vi "example_01_table_scrollbars.vi"() -> ()   [LabVIEW 2015, in "lv-pagination.lvlib"]
doc: "This example shows how to use both auto-sizing AND paging with a static data set that can be changed at will."
uses:
  lv-pagination.lvlib
  public/_controls/configuratin_resize.ctl
panel:
  in  "actual_fuzzy":bool
  in  "random":bool
  in  "configuration":T1=enum."all"
  in  "precision":i32=6
  out "configuration []":cluster{"width":u32, "height":u32}[](array[cluster])
  in  "rows":i32=100
  in  "columns":i32=20
  in  "auto_size":bool
  in  "load_column_width":bool
  in  "save_column_width":bool
  in  "sticky_column":i32=-1
  out "data":i32(listbox)=-1
  in  "horizontal":i32(c297)
  in  "vertical":i32(c297)
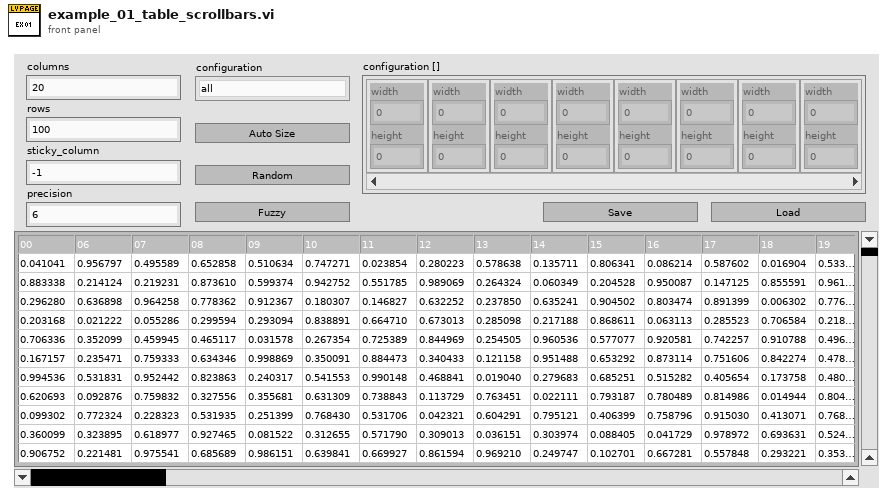
[diagram p1: front panel]
types:
  T1 = typedef "lv-pagination.lvlib/configuratin_resize.ctl" = enum16{"<resize_config>", "header", "contents", "all", "best_fit"}
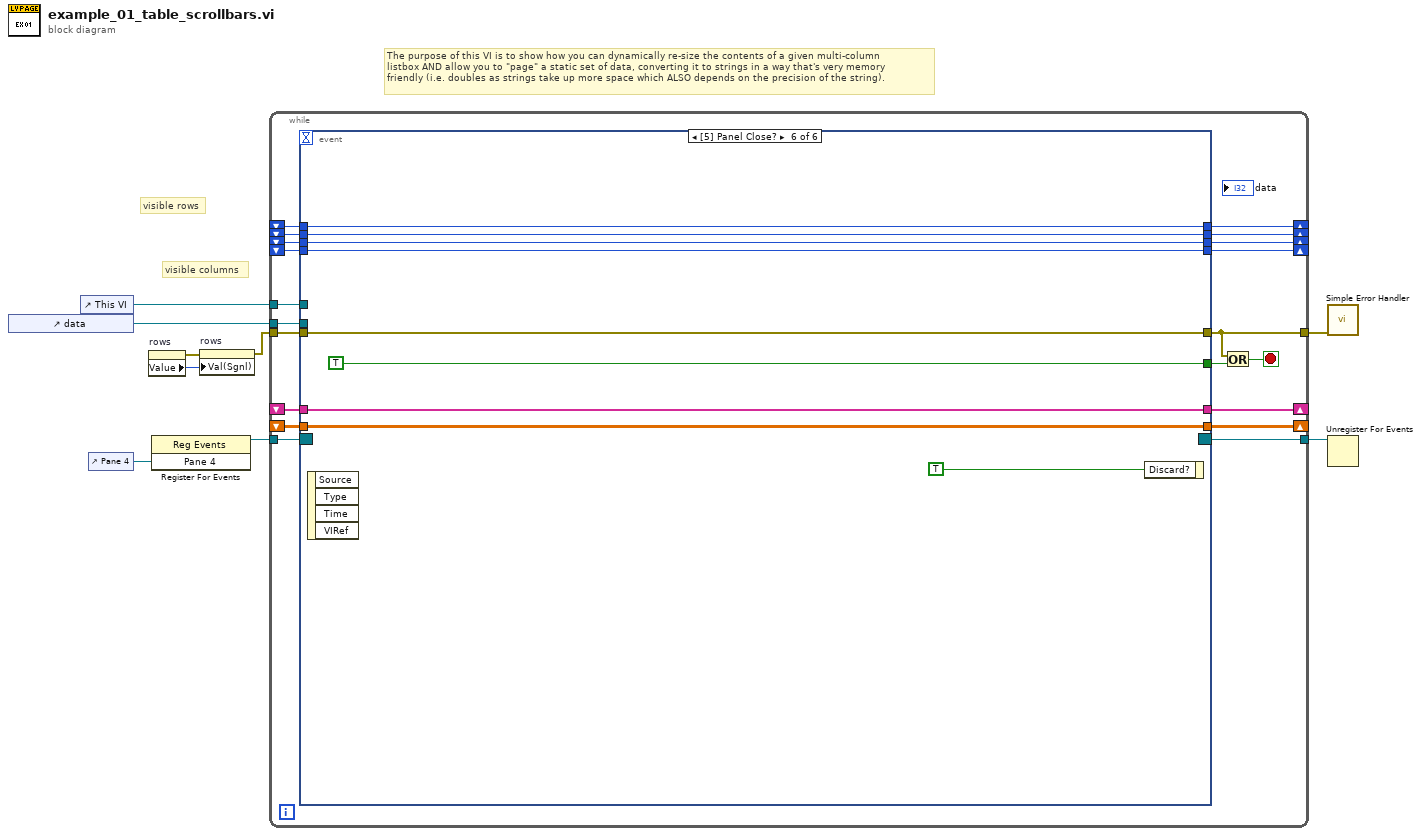
[diagram p0: block diagram]
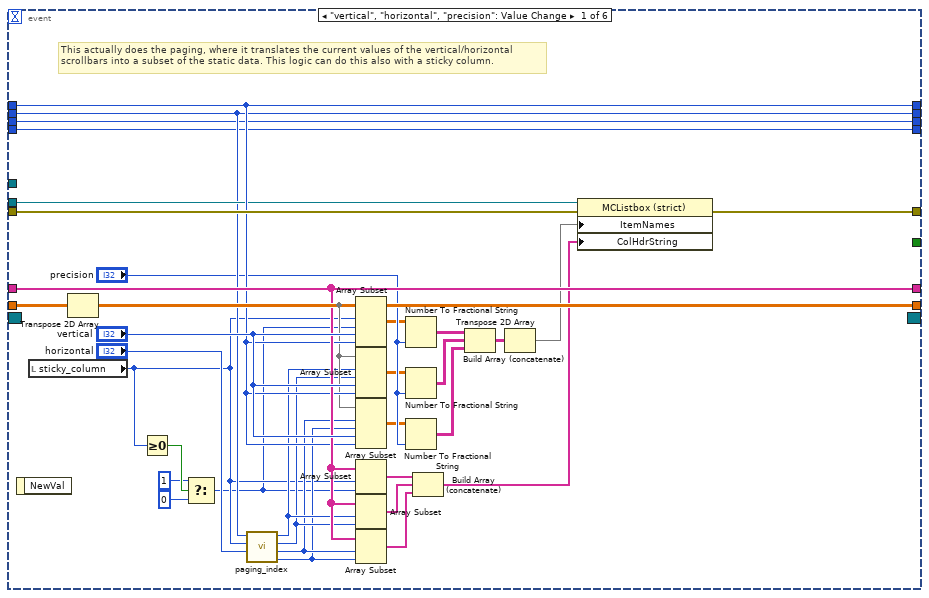
[diagram p2: hidden frame]
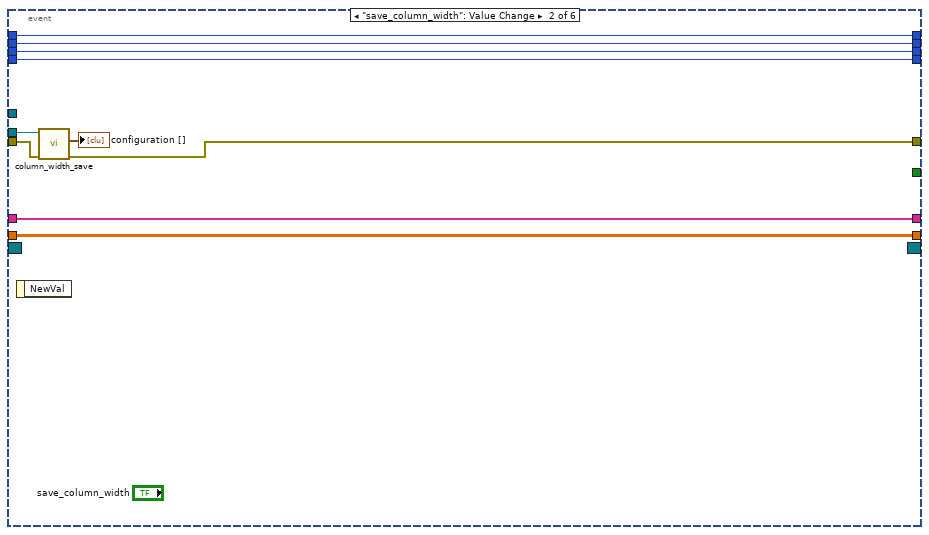
[diagram p3: hidden frame]
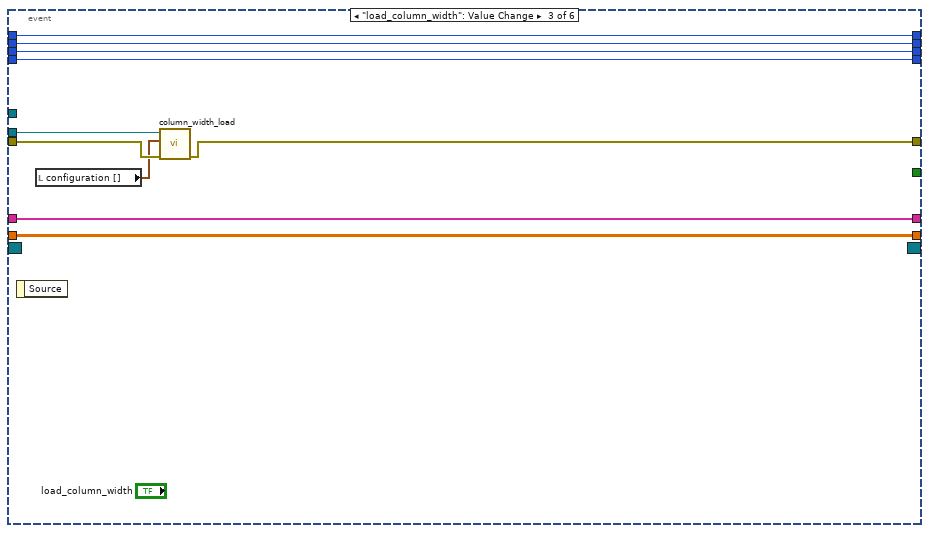
[diagram p4: hidden frame]
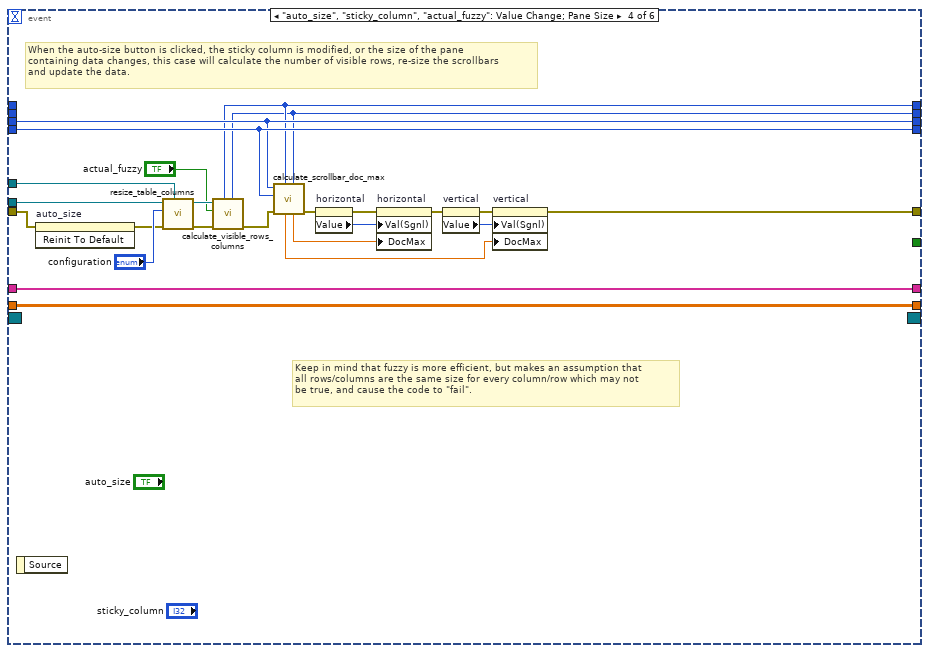
[diagram p5: hidden frame]
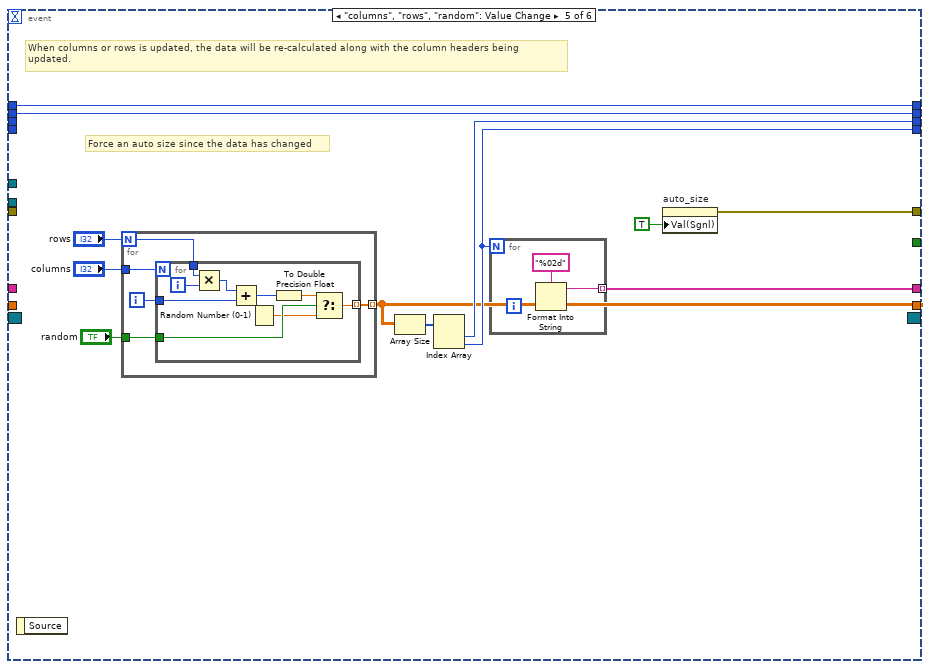
[diagram p6: hidden frame]
diagram:
  # "The purpose of this VI is to show how you can dynamically re-size the contents of a given multi-column\nlistbox AND allow you to \"page\" a static set of data, converting it to strings in a way that's very memory\nfriendly (i.e. doubles as strings take up more space which ALSO depends on the precision of the string)."
  # "visible columns"
  # "visible rows"
  n1 = control-ref of="data"() -> (w4:refnum<vi>)
  n2 = control-ref of="This VI"() -> (w5:refnum<vi>)
  n3 = control-ref of="Pane 4"() -> (w8:refnum<vi>)
  n4 = property on="rows" class="DigNum (strict)"() -> (error out=w1:errorcluster, "Value"=w3:i32)  [unwired: 2 in, 1 out]
  n5 = register-events(w8) -> (reference out=w7:refnum<event-registration>)  [unwired: 2 in, 1 out]
  n6 = property on="rows" class="DigNum (strict)"(error in=w1, "Val(Sgnl)"=w3) -> (error out=w2:errorcluster)  [unwired: 1 in, 1 out]
  n7 = while {
    shift-right: [w25] -> _
    shift-left: _ -> [w28]
    tunnel: w4 -> [w23]
    shift-right: [w21] -> _
    shift-left: _ -> [w22]
    tunnel: w2 -> [w27]
    tunnel: [w19] -> w9
    tunnel: w7 -> [w16]
    tunnel: [w15] -> w6
    tunnel: w5 -> [w14]
    shift-right: [w13] -> _
    shift-left: _ -> [w29]
    shift-right: [w12] -> _
    shift-left: _ -> [w26]
    shift-right: [w11] -> _
    shift-left: _ -> [w24]
    shift-right: [w10] -> _
    shift-left: _ -> [w20]
    stop <- w18 stop-if-true
    n8 = event shown="[5] Panel Close?" {
      selector: w16 -> [_ _ _ _ _ _]
      dyn-events: [_ _ _ _ _ _] -> w15
      timeout: _ -> [_ _ _ _ _ _]
      tunnel: w29 -> [w62 w67 w77 w97 _ w140]
      tunnel: w28 -> [w59 w70 w79 _ w118 w144]
      tunnel: w27 -> [w63 w73 w83 w95 _ w141]
      tunnel: w26 -> [w60 w66 w76 w96 _ w139]
      tunnel: [w59 w70 w79 w98 w118 w144] -> w25
      tunnel: w24 -> [w51 w65 w75 w99 _ w138]
      tunnel: [w30 w72 w80 w105 w107 w141] -> w19
      tunnel: w23 -> [w57 w71 w81 w103 _ _]
      tunnel: w22 -> [w56 w69 w78 _ w117 w143]
      tunnel: [w56 w69 w78 w93 w117 w143] -> w21
      tunnel: w20 -> [w50 w64 w74 w100 _ w137]
      tunnel: [_ _ _ _ _ TRUE] -> w17
      tunnel: w14 -> [_ _ _ w104 _ _]
      tunnel: [w62 w67 w77 w97 w111 w140] -> w13
      tunnel: [w60 w66 w76 w96 w110 w139] -> w12
      tunnel: [w51 w65 w75 w99 w114 w138] -> w11
      tunnel: [w50 w64 w74 w100 w113 w137] -> w10
      event "vertical", "horizontal", "precision": Value Change {
        # "This actually does the paging, where it translates the current values of the vertical/horizontal\nscrollbars into a subset of the static data. This logic can do this also with a sticky column."
        n9 = event-data() -> ()  [unwired: 1 in, 1 out]
        n10 = local read "sticky_column"() -> (w35:i32)
        n11 = Transpose 2D Array(2D array=w62) -> (transposed array=w52:dbl[][])
        n12 = Greater Or Equal To 0?(x=w35) -> (x >= 0?=w34:bool)
        n13 = Select(t=1 ("length"), s=w34, f=0 ("length")) -> (s? t:f=w31:i32)
        n14 = call "paging_index.vi"("horizontal_scrollbar"="horizontal", "sticky_column"=w35, "visible_columns"=w56) -> ("post_sticky_length"=w46:i32, "post_sticky_index"=w47:i32, "pre_sticky_length"=w48:i32, "pre_sticky_index"=w49:i32)  [unwired: 5 in]
        n15 = Array Subset(array=w52, index (row)=w35, length (row)=w31, index (col)="vertical", length (col)=w59) -> (w38:dbl[][])
        n16 = Array Subset(array=w52, index (row)=w49, length (row)=w48, index (col)="vertical", length (col)=w59) -> (w37:dbl[][])
        n17 = Array Subset(array=w52, index (row)=w47, length (row)=w46, index (col)="vertical", length (col)=w59) -> (w36:dbl[][])
        n18 = Array Subset(array=w60, index=w35, length=w31) -> (w45:string[])
        n19 = Array Subset(array=w60, index=w49, length=w48) -> (w44:string[])
        n20 = Array Subset(array=w60, index=w47, length=w46) -> (w43:string[])
        n21 = Number To Fractional String(number=w38, precision (6)="precision") -> (F-format string=w39:string[][])  [unwired: 2 in]
        n22 = Number To Fractional String(number=w37, precision (6)="precision") -> (F-format string=w41:string[][])  [unwired: 2 in]
        n23 = Number To Fractional String(number=w36, precision (6)="precision") -> (F-format string=w42:string[][])  [unwired: 2 in]
        n24 = Build Array (concatenate)(w45, w44, w43) -> (w55:string[])
        n25 = Build Array (concatenate)(w39, w41, w42) -> (w40:string[][])
        n26 = Transpose 2D Array(2D array=w40) -> (transposed array=w53:string[][])
        n27 = property on="Property Node" class="MCListbox (strict)"(reference=w57, error in=w63, "ItemNames"=w53, "ColHdrString"=w55) -> (error out=w30:errorcluster)  [unwired: 1 out]
      }
      event "save_column_width": Value Change {
        n28 = event-data() -> ()  [unwired: 1 in, 1 out]
        n29 = call "column_width_save.vi"("error in (no error)"=w73, "listbox_reference"=w71) -> ("error out"=w72:errorcluster, "configuration []"=→"configuration []":cluster{"width":u32, "height":u32}[])  [unwired: 8 in]
      }
      event "load_column_width": Value Change {
        n30 = event-data() -> ()  [unwired: 1 in, 1 out]
        n31 = local read "configuration []"() -> (w82:cluster{"width":u32, "height":u32}[])
        n32 = call "column_width_load.vi"("error in (no error)"=w83, "configuration []"=w82, "listbox_reference"=w81) -> ("error out"=w80:errorcluster)  [unwired: 8 in]
      }
      event "auto_size", "sticky_column", "actual_fuzzy": Value Change; Pane Size {
        # "Keep in mind that fuzzy is more efficient, but makes an assumption that\nall rows/columns are the same size for every column/row which may not\nbe true, and cause the code to \"fail\"."
        # "When the auto-size button is clicked, the sticky column is modified, or the size of the pane\ncontaining data changes, this case will calculate the number of visible rows, re-size the scrollbars\nand update the data."
        n33 = event-data() -> ()  [unwired: 1 in, 1 out]
        n34 = invoke on="auto_size" class="Bool (strict)" method="Reinit To Default"(error in=w95) -> (error out=w94:errorcluster)  [unwired: 2 in, 2 out]
        n35 = call "resize_table_columns.vi"("vi_reference"=w104, "error in (no error)"=w94, "configuration"="configuration", "listbox_reference"=w103) -> ("error out"=w102:errorcluster)  [unwired: 7 in]
        n36 = call "calculate_visible_rows_columns.vi"("error in (no error)"=w102, "actual"="actual_fuzzy", "listbox_reference"=w103) -> ("error out"=w101:errorcluster, "visible_columns"=w93:i32, "visible_rows"=w98:i32)  [unwired: 6 in]
        n37 = call "calculate_scrollbar_doc_max.vi"("visible_columns"=w93, "visible_rows"=w98, "error in (no error)"=w101, "data_columns"=w100, "data_rows"=w99) -> ("error out"=w91:errorcluster, "horizontal"=w88:dbl, "vertical"=w89:dbl)  [unwired: 4 in]
        n38 = property on="horizontal" class="Scroll (strict)"(error in=w91) -> (error out=w87:errorcluster, "Value"=w84:i32)  [unwired: 1 in, 1 out]
        n39 = property on="horizontal" class="Scroll (strict)"(error in=w87, "Val(Sgnl)"=w84, "DocMax"=w88) -> (error out=w90:errorcluster)  [unwired: 1 in, 1 out]
        n40 = property on="vertical" class="Scroll (strict)"(error in=w90) -> (error out=w86:errorcluster, "Value"=w85:i32)  [unwired: 1 in, 1 out]
        n41 = property on="vertical" class="Scroll (strict)"(error in=w86, "Val(Sgnl)"=w85, "DocMax"=w89) -> (error out=w105:errorcluster)  [unwired: 1 in, 1 out]
      }
      event "columns", "rows", "random": Value Change {
        # "Force an auto size since the data has changed"
        # "When columns or rows is updated, the data will be re-calculated along with the column headers being\nupdated."
        n42 = event-data() -> ()  [unwired: 1 in, 1 out]
        n43 = for {
          N: "rows" -> [w122]
          tunnel: [w126] -> w111 mode=indexing
          tunnel: "columns" -> [w125]
          tunnel: "random" -> [w123]
          i -> [w124]
          n44 = for {
            N: w125 -> [_]
            tunnel: [w133] -> w126 mode=indexing
            tunnel: w124 -> [w135]
            tunnel: w123 -> [w132]
            tunnel: w122 -> [w129]
            i -> [w131]
            n45 = Multiply(x=w129, y=w131) -> (x*y=w130:i32)
            n46 = Add(x=w130, y=w135) -> (x+y=w134:i32)
            n47 = Random Number (0-1)() -> (number: 0 to 1=w128:dbl)
            n48 = To Double Precision Float(number=w134) -> (double precision float=w127:dbl)
            n49 = Select(t=w127, s=w132, f=w128) -> (s? t:f=w133:dbl)
          }
        }
        n50 = Array Size(array=w111) -> (size(s)=w115:i32[])
        n51 = Index Array(array=w115) -> (element #1=w114:i32, element #2=w113:i32)  [unwired: 2 in]
        n52 = for {
          N: w113 -> [_]
          tunnel: [w120] -> w110 mode=indexing
          i -> [w119]
          n53 = Format Into String(format string="%02d", w119) -> (resulting string=w120:string)  [unwired: 2 in, 1 out]
        }
        n54 = property on="auto_size" class="Bool (strict)"("Val(Sgnl)"=TRUE) -> (error out=w107:errorcluster)  [unwired: 2 in, 1 out]
      }
      event Panel Close? {
        n55 = event-data() -> ()  [unwired: 1 in, 4 out]
        n56 = event-data("Discard?"=TRUE) -> ()  [unwired: 1 in, 1 out]
      }
    }
    n57 = Or(x=w19, y=w17) -> (x .or. y?=w18:bool)
  }
  n58 = call <vilib>:"Simple Error Handler.vi"("error in (no error)"=w9) -> ()  [unwired: 4 in, 5 out]
  n59 = Unregister For Events(event registration refnum=w6) -> ()  [unwired: 1 in, 1 out]
